vi "1D_Jacobi_eigenvalue_algorithm_v7.vi"() -> ()   [LabVIEW 2020]
uses:
  <vilib>/Analysis/baseanly.llb/Real A x B.vi
  <vilib>/Analysis/baseanly.llb/Mean (DBL).vi
  <vilib>/Analysis/Matrix/Numeric/Conversions/Array To Matrix - RA2.vi
  <vilib>/Analysis/Matrix/Numeric/Conversions/Matrix To Array - RM.vi
  <vilib>/Analysis/7linalg.llb/Real Eigenvalues and Vectors.vi
  <vilib>/Analysis/Matrix/NI_Matrix.lvlib
  <vilib>/Analysis/NI_AALBase.lvlib
  <vilib>/Analysis/NI_AALPro.lvlib
panel:
  out "percent error":dbl
  out "FPGA Jacobi eigenvalue":sgl[](array[numeric])
  in  "Number of Rotations":i32=100
  out "A":dbl[][](array[numeric])
  out "LabVIEW eigvals":dbl[](array[numeric])
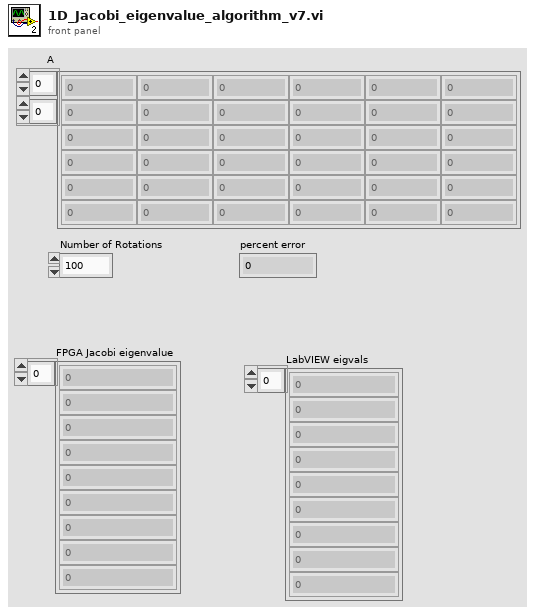
[diagram p1: front panel]
types:
  T1 = typedef "NI_Matrix.lvlib/RealMatrix.ctl" = dbl[][]
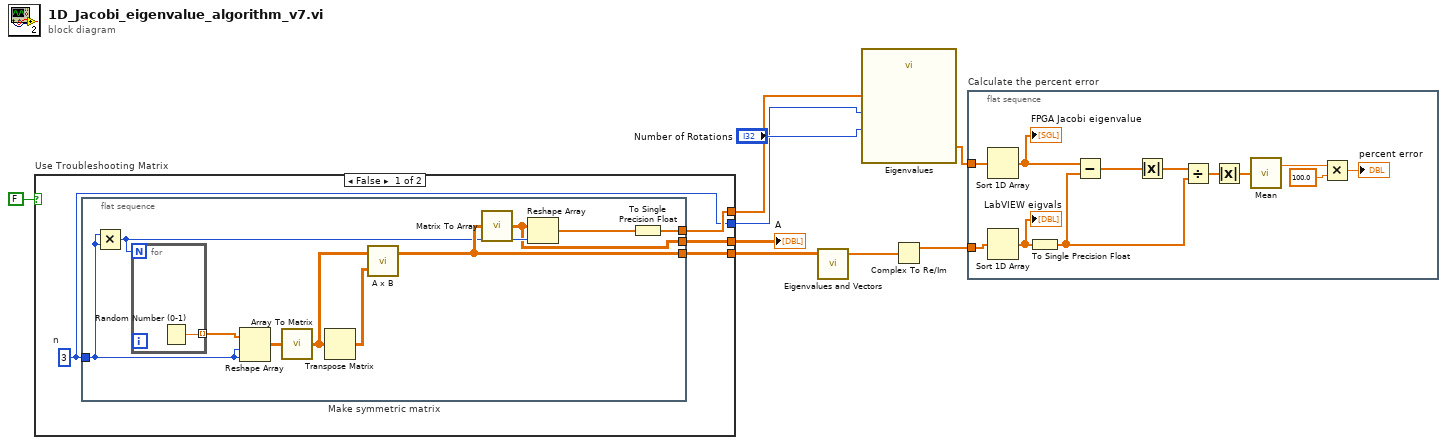
[diagram p0: block diagram]
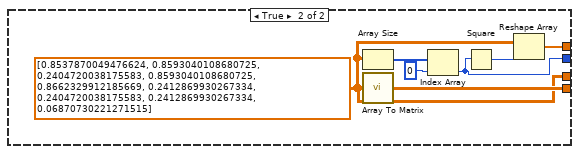
[diagram p2: hidden frame]
diagram:
  n1 = case "Use Troubleshooting Matrix" shown="False" FALSE {
    tunnel: [w12 w31] -> w8
    tunnel: [w13 w30] -> w6
    tunnel: [w11 w28] -> w3
    tunnel: [w10 w25] -> w1
    frame False {
      w10 = 3  # n
      n2 = flat-sequence "Make symmetric matrix" {
        tunnel: [w19] -> w12
        tunnel: [w17] -> w13
        tunnel: [w15] -> w11
        tunnel: w10 -> [w14]
        frame #0 {
          n3 = Multiply(x=w14, y=w14) -> (x*y=w16:i32)
          n4 = for {
            N: w16 -> [_]
            tunnel: [w24] -> w23 mode=indexing
            n5 = Random Number (0-1)() -> (number: 0 to 1=w24:dbl)
          }
          n6 = Reshape Array(w23, w14, w14) -> (w22:dbl[][])
          n7 = call-poly <vilib>:"Array To Matrix.vi"("Real 2D Array"=w22) -> ("Real Matrix"=w21:T1)
          n8 = Transpose Matrix(1:w21) -> (0:w20:T1)
          n9 = call-poly <vilib>:"A x B.vi"("B"=w20, "A"=w21) -> ("A x B"=w19:T1)  [unwired: 1 out]
          n10 = call-poly <vilib>:"Matrix To Array.vi"("Real Matrix"=w19) -> ("Real 2D Array"=w15:dbl[][])
          n11 = Reshape Array(w15, w16) -> (w18:dbl[])
          n12 = To Single Precision Float(number=w18) -> (single precision float=w17:sgl[])
        }
      }
    }
    frame True {
      w28 = sgl[][] [[0.853787, 0.859304, 0.240472], [0.859304, 0.866233, 0.241287], [0.240472, 0.241287, 0.0687073]]
      n13 = Array Size(array=w28) -> (size(s)=w27:i32[])
      n14 = call-poly <vilib>:"Array To Matrix.vi"("Real 2D Array"=w28) -> ("Real Matrix"=w31:T1)
      n15 = Index Array(array=w27, index=0) -> (element=w25:i32)
      n16 = Square(x=w25) -> (x^2=w29:i32)
      n17 = Reshape Array(w28, w29) -> (w30:sgl[])
    }
  }
  "A" <- w3
  n18 = call-poly <vilib>:"Eigenvalues and Vectors.vi"("Input Matrix"=w8) -> ("Eigenvalues"=w9:cdb[])  [unwired: 2 in, 2 out]
  n19 = call "Eigenvalues.vi"("n"=w1, "Number of Rotations"="Number of Rotations", "A"=w6) -> ("eigenvalues"=w5:sgl[])
  n20 = Complex To Re/Im(x + iy=w9) -> (x=w4:dbl[])  [unwired: 1 out]
  n21 = flat-sequence "Calculate the percent error" {
    tunnel: w5 -> [w43]
    tunnel: w4 -> [w42]
    frame #0 {
      n22 = Sort 1D Array(array=w43) -> (sorted array=w40:sgl[])
      "FPGA Jacobi eigenvalue" <- w40
      n23 = Sort 1D Array(array=w42) -> (sorted array=w41:dbl[])
      "LabVIEW eigvals" <- w41
      n24 = To Single Precision Float(number=w41) -> (single precision float=w37:sgl[])
      n25 = Subtract(x=w40, y=w37) -> (x-y=w39:sgl[])
      n26 = Absolute Value(x=w39) -> (abs(x)=w38:sgl[])
      n27 = Divide(x=w38, y=w37) -> (x/y=w36:sgl[])
      n28 = Absolute Value(x=w36) -> (abs(x)=w35:sgl[])
      n29 = call-poly <vilib>:"Mean.vi"("X"=w35) -> ("mean"=w34:dbl)  [unwired: 1 out]
      n30 = Multiply(x=w34, y=100.0) -> (x*y=→"percent error":dbl)
    }
  }
